vi "Get RFSG Power.vi"(0 "Path in":refnum<class "Scalar Path.lvclass">, 11 "error in (no error)":errorcluster) -> (4 "Path out":refnum<class "Scalar Path.lvclass">, 6 "Power Level (dBm)":dbl, 15 "error out":errorcluster)   [LabVIEW 2023, in "RFFixtureCharact.Public.lvlib" / "Scalar Path.lvclass"]
uses:
  Scalar Path.lvclass
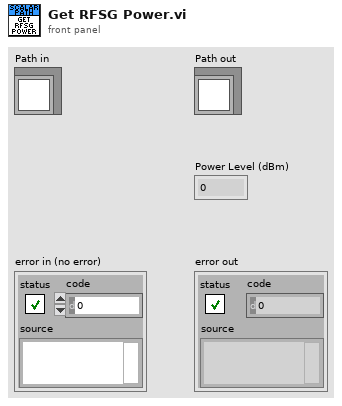
[diagram p1: front panel]
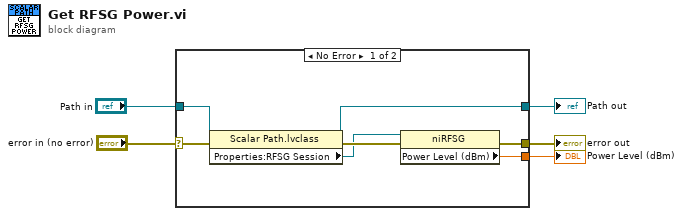
[diagram p0: block diagram]
diagram:
  n1 = case shown="No Error" "error in (no error)" {
    selector: "error in (no error)" -> [w11 w14]
    tunnel: [w8 w14] -> w4
    tunnel: [w10 w13] -> w1
    tunnel: "Path in" -> [w12 w13]
    tunnel: [w7 _] -> w3
    frame No Error {
      n2 = property class="Scalar Path.lvclass"(reference=w12, error in=w11) -> (reference out=w10:refnum<class "Scalar Path.lvclass">, error out=w9:errorcluster, "Properties:RFSG Session"=w6:refnum<k15>)
      n3 = property class="niRFSG"(reference=w6, error in=w9) -> (error out=w8:errorcluster, "Power Level (dBm)"=w7:dbl)  [unwired: 1 out]
    }
    frame Error {
    }
  }
  "error out" <- w4
  "Power Level (dBm)" <- w3
  "Path out" <- w1
